vi "PC send voltage and resistance when in local mode.vi"(5 "Resistance":dbl, 9 "Voltage":dbl, 11 "error in (no error)":errorcluster) -> (15 "error out":errorcluster)   [LabVIEW 2011]
uses:
  High Level/PCP High Level Commands.ctl
  Application Structure/QSM State List.ctl
  High Level/PCP High Level Telegram.ctl
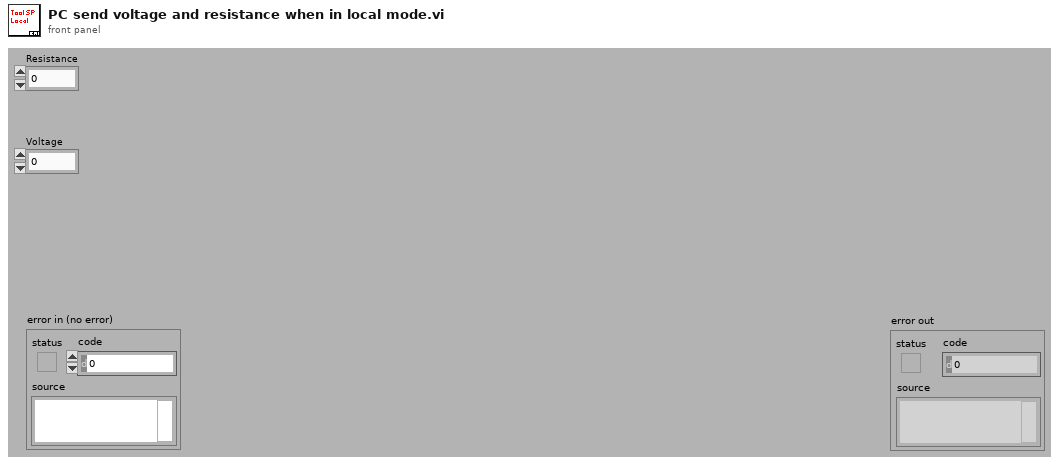
[diagram p1: front panel]
types:
  T1 = typedef "PCP High Level Commands.ctl" = enum16{"HVPSU HV ON", "HVPSU HV OFF", "PCP PC", "PCP Local", "Update Motor Voltage", "Update Cable Resistance", "Final Motor Voltage", "Final Resistance"}
  T2 = typedef "PCP High Level Telegram.ctl" = cluster{"PCP":T1, "SP":dbl}
  T3 = typedef "QSM State List.ctl" = enum16{"Idle", "Init <<<Start>>>", "Init Reg Controlers", "Init Stroker Ref FGV", "Init Driller Ref FGV", "Init Tractor Ref FGV", "Init All loops", "Init Mem Ctls", "Init GUI", "Init<<<End>>>", "Show options", "Options updated", "Show User Dialog", "User Updated", "Show About", "Show Help", "Debug Visibility", "End Application", "Mem Ctls", "Mem Graphs", "Post", "-------------", "Dialog Common Analog", "Chart Init", "Chart Var Selector Rings init", "Chart Read Settings from INI", "Chart Clear", "Chart Selection Changed", "Chart Time Changed", "Graph Dialog Show", "Annotation, New", "Annotation Created", "PCP CMD", "Show Welcome screen", "Dialog Tool analog", "Update PCP resistance", "Tool CMD", "Chart single autoscale", "Tool connenction state", "Show detailed view", "Sequences updated", "Show stroker wizard", "Change tool", "Reset Telemetry", "Update control units", "Stop Logging", "Start New Loggfile", "Log Init", "Copy INI files"}
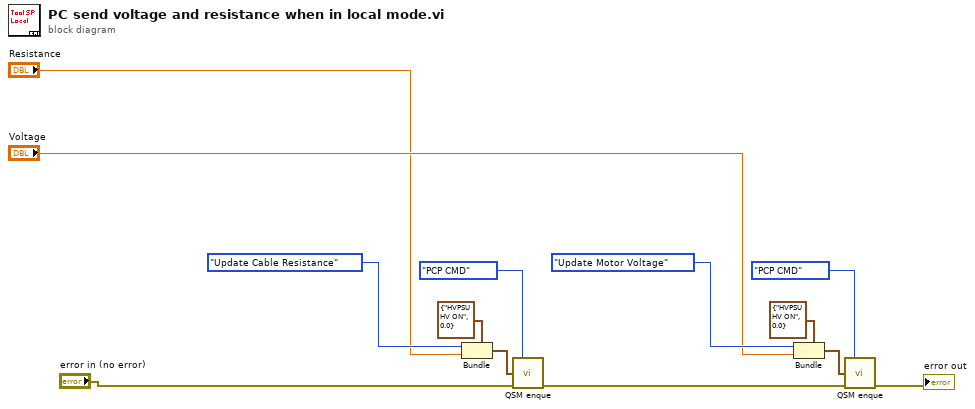
[diagram p0: block diagram]
diagram:
  n1 = Bundle(cluster=T2 {"PCP"=enum."HVPSU HV ON", "SP"=0.0} ("PCP beskjed"), "PCP"=PCP_High_Level_Commands."Update Cable Resistance", "SP"="Resistance") -> (w7:T2)
  n2 = call "QSM enque.vi"("State"=QSM_State_List."PCP CMD", "Value"=w7, "error in"="error in (no error)") -> ("error out"=w2:errorcluster)  [unwired: 12 in]
  n3 = Bundle(cluster=T2 {"PCP"=enum."HVPSU HV ON", "SP"=0.0} ("PCP beskjed"), "PCP"=PCP_High_Level_Commands."Update Motor Voltage", "SP"="Voltage") -> (w11:T2)
  n4 = call "QSM enque.vi"("State"=QSM_State_List."PCP CMD", "Value"=w11, "error in"=w2) -> ("error out"=→"error out":errorcluster)  [unwired: 12 in]
